vi "2MotorFinalNoKinematics (1).vi"() -> ()   [LabVIEW 2017]
uses:
  <vilib>/Platform/TimedLoop/XDataNode/timing_clust.ctl
  <vilib>/Platform/TimedLoop/XDataNode/nitl_modes.ctl
  <vilib>/Platform/TimedLoop/XDataNode/wakeup.ctl
  <vilib>/platform/TimedLoop/XDataNode/XDataNode.xnode
  <vilib>/Platform/TimedLoop/XDataNode/XDNodeRunTimeDep.lvlib
panel:
  in  "Kd 2":dbl(slide) scale=0.0..0.5
  in  "Ki 2":dbl(slide) scale=0.0..10.0
  in  "Kp 2":dbl(slide) scale=0.01..50.0
  in  "Manual\nControl":bool
  in  "X 2":dbl
  in  "Y 2":dbl
  out "Q2 (Top Motor)":dbl
  out "Q1":dbl
  in  "stop":bool
  out "Waveform Chart 2":cluster{"Numeric":dbl, "Ref 2":dbl}(graph)
  out "Waveform Chart":cluster{"Numeric":dbl, "Ref 1":dbl}(graph)
  out "Analog 2":dbl(knob) scale=0.0..5.0
  out "Analog 1":dbl(knob) scale=0.0..5.0
  out "Pos 2":dbl(knob) scale=0.0..360.0
  out "Pos 1":dbl(knob) scale=0.0..360.0
  in  "Initialize Int 2":bool
  in  "Initialize Int 1":bool
  in  "Q 2":dbl(slide) scale=-180.0..180.0
  in  "Q 1":dbl(slide) scale=-180.0..180.0
  in  "Kd":dbl(slide) scale=0.0..0.5
  in  "Ki":dbl(slide) scale=0.0..10.0
  in  "Kp":dbl(slide) scale=0.01..50.0
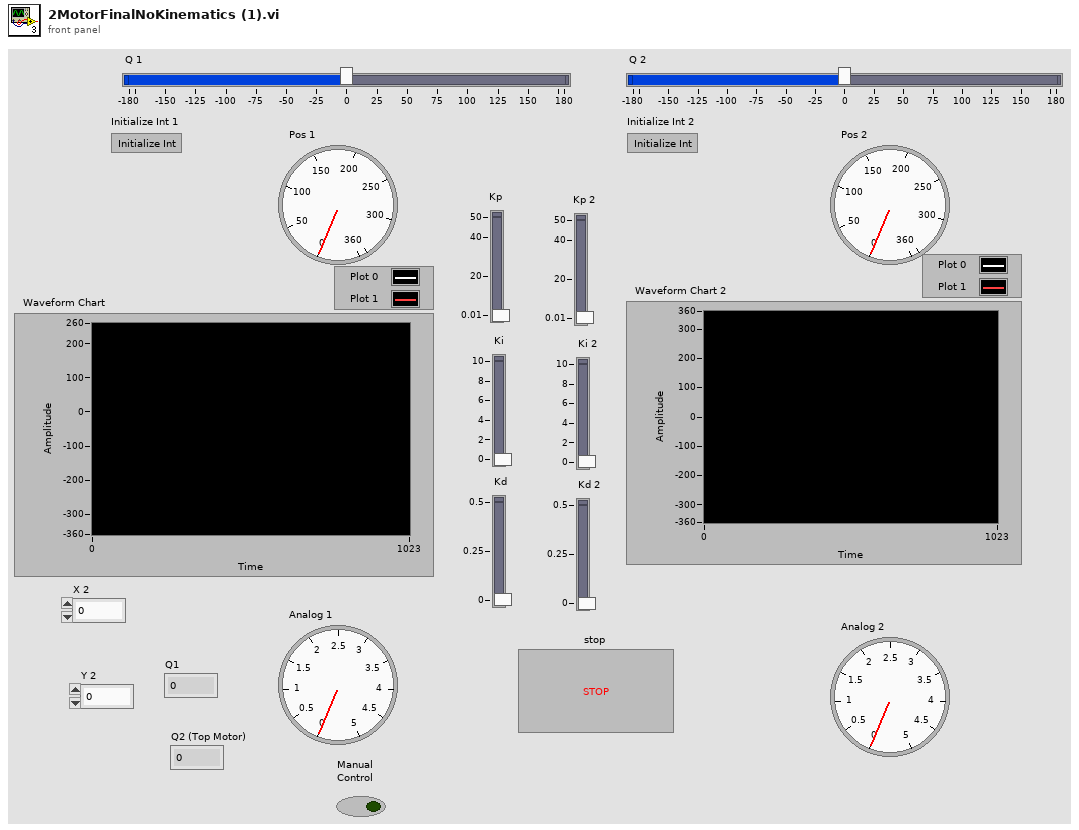
[diagram p1: front panel]
types:
  T1 = typedef "XDNodeRunTimeDep.lvlib/timing_clust.ctl" = cluster{"Expected End [f-1]":u64, "Actual End [f-1]":u64, "Finished Late? [f-1]":bool, "Expected End [i-1]":u64, "Actual End [i-1]":u64, "Finished Late? [i-1]":bool, "Expected Start [i]":u64, "Actual Start [i]":u64, "Expected Start [f]":u64, "Actual Start [f]":u64, "Source Name":string, "Structure Name":string, "Period":i64, "Deadline":i64, "Offset":i64, "Start":i64, "Priority":i32, "Timeout":i32, "Mode":T2, "Wakeup Reason":T3, "Error":errorcluster, "Source Type":string, "Secondary Source Type":string, "Global End Time":u64, "Global Start Time":u64, "Frame Duration":u64, "Iteration Duration":u64, "Assigned CPU":i32, "I/O Scan Engine Mode":u32}
  T2 = typedef "XDNodeRunTimeDep.lvlib/nitl_modes.ctl" = enum32{"No Change", "Process missed periods, maintain original phase", "Discard missed periods, maintain original phase", "Process missed periods, ignore original phase", "Discard missed periods, ignore original phase"}
  T3 = typedef "XDNodeRunTimeDep.lvlib/wakeup.ctl" = enum32{"Normal", "Aborted", "Asynchronous wakeup", "Timing source error", "Timed loop error", "Timeout"}
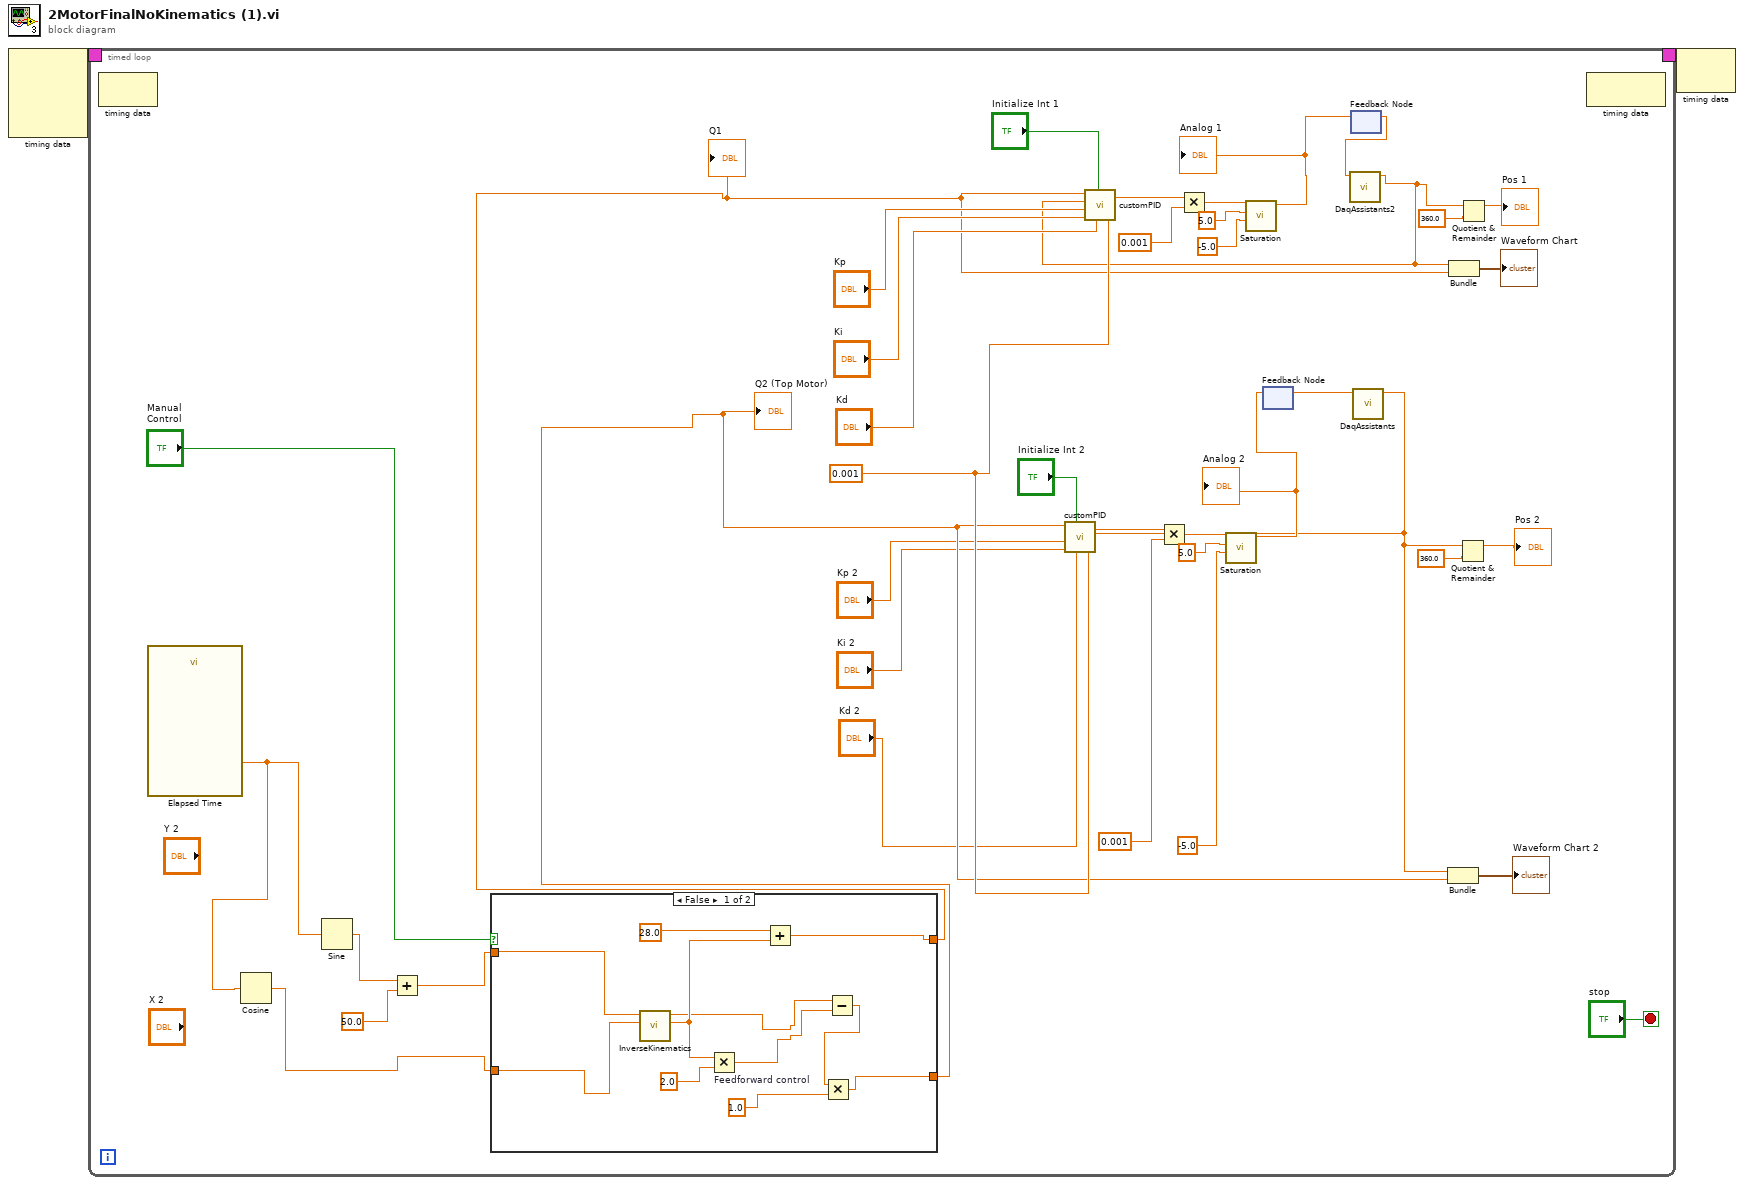
[diagram p0: block diagram]
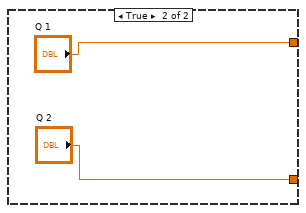
[diagram p2: hidden frame]
diagram:
  n1 = node-c288() -> (w2:T1)  [unwired: 4 in]
  n2 = timed-loop {
    timing: w2 -> [_]
    timing-out: [_] -> w1
    stop <- "stop" stop-if-true
    w20 = 0.001
    n3 = node-c288() -> ()  [unwired: 1 in, 1 out]
    n4 = call "Elapsed Time"() -> ("Elapsed Time (s)"=w7:dbl)  [unwired: 12 in, 7 out]
    n5 = Cosine(x=w7) -> (cos(x)=w4:dbl)
    n6 = Sine(x=w7) -> (sin(x)=w5:dbl)
    n7 = Add(x=w5, y=50.0) -> (x+y=w6:dbl)
    n8 = case shown="False" "Manual\nControl" {
      tunnel: [w48 "Q 1"] -> w12
      tunnel: [w50 "Q 2"] -> w11
      tunnel: w6 -> [w53 _]
      tunnel: w4 -> [w52 _]
      frame False {
        n9 = call "InverseKinematics.vi"("X"=w52, "Y"=w53) -> ("Q2"=w47:dbl, "Q1"=w45:dbl)  [unwired: 8 in]
        n10 = Multiply "Feedforward control"(x=w47, y=2.0) -> (x*y=w44:dbl)
        n11 = Add(x=28.0, y=w47) -> (x+y=w48:dbl)
        n12 = Subtract(x=w45, y=w44) -> (x-y=w43:dbl)
        n13 = Multiply(x=w43, y=1.0) -> (x*y=w50:dbl)
      }
      frame True {
      }
    }
    "Q1" <- w12
    "Q2 (Top Motor)" <- w11
    n14 = feedback #1() -> (w18:dbl)  [unwired: 1 in]
    n15 = feedback #2() -> (w14:dbl)  [unwired: 1 in]
    n16 = call "DaqAssistants2.vi"("output"=w14) -> ("Numeric"=w16:dbl)  [unwired: 10 in]
    n17 = call "customPID.vi"("dt"=w20, "Kd"="Kd", "Initialize"="Initialize Int 1", "Ki"="Ki", "Kp"="Kp", "Measured"=w16, "Desired"=w12) -> ("Motor Input"=w41:dbl)
    n18 = Multiply(x=w41, y=0.001) -> (x*y=w40:dbl)
    n19 = call "Saturation.vi"("lower bound"=-5.0, "upper bound"=5.0, "input"=w40) -> ("output"=w15:dbl)  [unwired: 8 in]
    "Analog 1" <- w15
    n20 = feedback-in #2(w15) -> ()
    n21 = call "DaqAssistants.vi"("output"=w18) -> ("Numeric"=w17:dbl)  [unwired: 10 in]
    n22 = call "customPID.vi"("dt"=w20, "Kd"="Kd 2", "Initialize"="Initialize Int 2", "Ki"="Ki 2", "Kp"="Kp 2", "Measured"=w17, "Desired"=w11) -> ("Motor Input"=w30:dbl)
    n23 = Multiply(x=w30, y=0.001) -> (x*y=w29:dbl)
    n24 = call "Saturation.vi"("lower bound"=-5.0, "upper bound"=5.0, "input"=w29) -> ("output"=w19:dbl)  [unwired: 8 in]
    "Analog 2" <- w19
    n25 = feedback-in #1(w19) -> ()
    n26 = Bundle("Numeric"=w17, "Q 2"=w11) -> (→"Waveform Chart 2":cluster{"Numeric":dbl, "Q 2":dbl})  [unwired: 1 in]
    n27 = Bundle("Numeric"=w16, "Q 1"=w12) -> (→"Waveform Chart":cluster{"Numeric":dbl, "Q 1":dbl})  [unwired: 1 in]
    n28 = Quotient & Remainder(x=w17, y=360.0) -> (x-y*floor(x/y)=→"Pos 2":dbl)  [unwired: 1 out]
    n29 = Quotient & Remainder(x=w16, y=360.0) -> (x-y*floor(x/y)=→"Pos 1":dbl)  [unwired: 1 out]
    n30 = node-c288() -> ()  [unwired: 1 in, 1 out]
  }
  n31 = node-c288(w1) -> ()  [unwired: 1 out]
